vi "display_notifier.vi"() -> (0 "error out":errorcluster, 3 "Notifier out":refnum<notifier>)   [LabVIEW 2013]
uses:
  type_defs/display_update.ctl
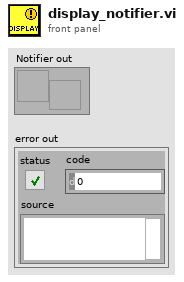
[diagram p1: front panel]
types:
  T1 = typedef "display_update.ctl" = enum16{"UPDATE"}
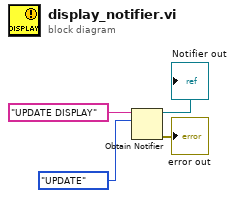
[diagram p0: block diagram]
diagram:
  n1 = Obtain Notifier(name (unnamed)="UPDATE DISPLAY", notification data type=display_update."UPDATE") -> (notifier out=→"Notifier out":refnum<notifier>, error out=→"error out":errorcluster)  [unwired: 2 in, 1 out]
